vi "TDS_NewConfigurationNumber.vi"(8 "error in (no error)":errorcluster) -> (0 "error out":errorcluster, 2 "Canceled?":bool, 3 "TDS.NewConfigurationRefOUT":string)   [LabVIEW 2020]
panel:
  in  "Scope.NewConfigRef.Cancel":bool
  in  "Scope.NewConfigRef.OK":bool
  in  "TDS.NewConfigurationRef":string
  # "Please enter new Scope configuration reference\n(limited to 7 characters)"
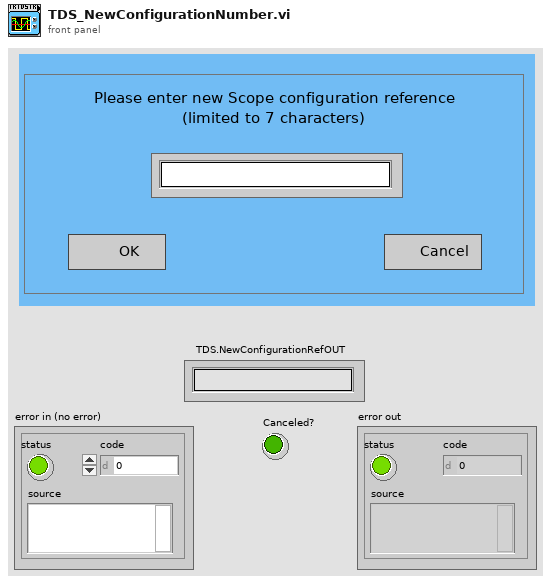
[diagram p1: front panel]
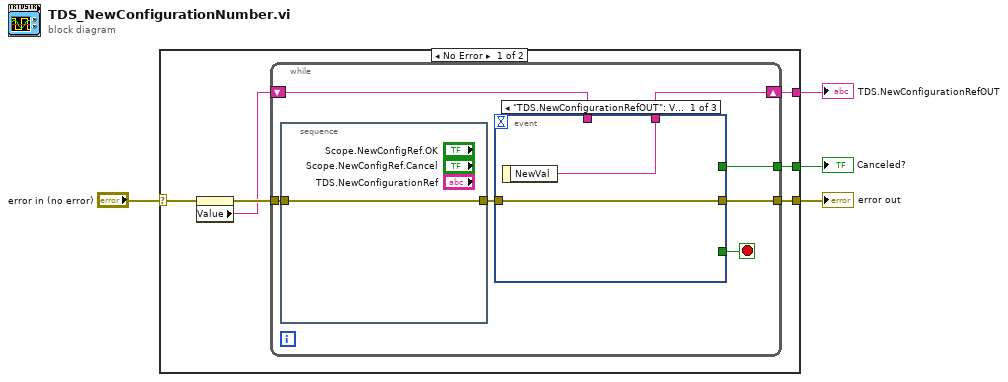
[diagram p0: block diagram]
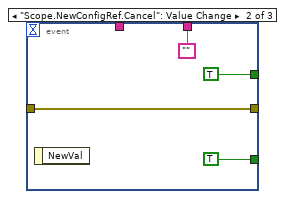
[diagram p2: hidden frame]
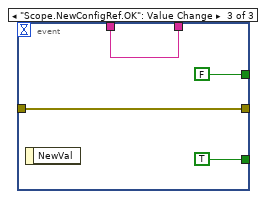
[diagram p3: hidden frame]
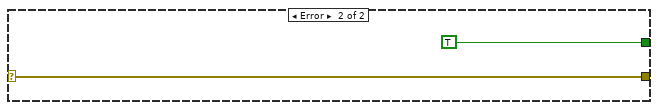
[diagram p4: hidden frame]
diagram:
  n1 = case shown="No Error" "error in (no error)" {
    selector: "error in (no error)" -> [w7 w30]
    tunnel: [w10 w30] -> w3
    tunnel: [w9 _] -> w2
    tunnel: [w8 TRUE] -> w1
    frame No Error {
      n2 = property on="TDS.NewConfigurationRef" class="Str"(error in=w7) -> (error out=w6:errorcluster, "Value"=w5:string)  [unwired: 1 in, 1 out]
      n3 = while {
        tunnel: w6 -> [w17]
        shift-right: [w14] -> w9
        shift-left: w5 -> [w15]
        tunnel: [w13] -> w10
        tunnel: [w11] -> w8
        stop <- w12 stop-if-true
        n4 = stacked-sequence {
          tunnel: [w28] -> w16
          tunnel: w17 -> [w28]
          frame #0 {
          }
        }
        n5 = event shown="[0] \"TDS.NewConfigurationRefOUT\": Value Change" {
          selector: _ -> [_ _ _]
          dyn-events: _ -> [_ _ _]
          timeout: _ -> [_ _ _]
          tunnel: w16 -> [w18 w23 w27]
          tunnel: w15 -> [_ _ w24]
          tunnel: [w19 "" w24] -> w14
          tunnel: [w18 w23 w27] -> w13
          tunnel: [_ TRUE TRUE] -> w12
          tunnel: [_ TRUE FALSE] -> w11
          event "TDS.NewConfigurationRefOUT": Value Change {
            n6 = event-data() -> ("NewVal"=w19:string)  [unwired: 1 in]
          }
          event "Scope.NewConfigRef.Cancel": Value Change {
            n7 = event-data() -> ()  [unwired: 1 in, 1 out]
          }
          event "Scope.NewConfigRef.OK": Value Change {
            n8 = event-data() -> ()  [unwired: 1 in, 1 out]
          }
        }
      }
    }
    frame Error {
    }
  }
  "TDS.NewConfigurationRefOUT" <- w2
  "error out" <- w3
  "Canceled?" <- w1
